vi "Error Handling SubVI Example.vi"(8 "error in (no error)":errorcluster, 10 "Frequency":dbl=10.1, 11 "Amplitude":dbl=1.0) -> (0 "error out":errorcluster, 3 "Waveform":waveform(dbl))   [LabVIEW 2015]
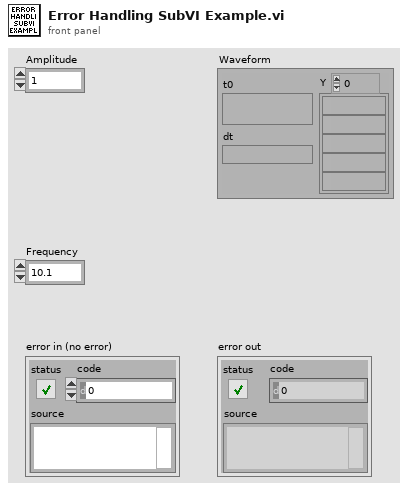
[diagram p1: front panel]
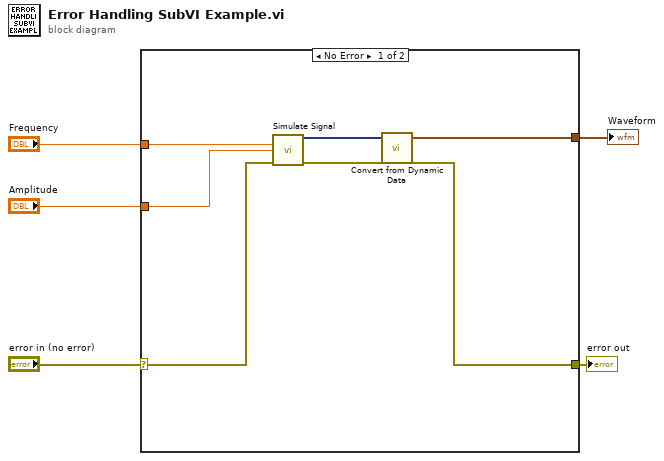
[diagram p0: block diagram]
diagram:
  n1 = case shown="No Error" "error in (no error)" {
    selector: "error in (no error)" -> [w10 w12]
    tunnel: [w9 w12] -> w4
    tunnel: "Frequency" -> [w8 _]
    tunnel: "Amplitude" -> [w7 _]
    tunnel: [w6 _] -> w1
    frame No Error {
      n2 = call "Simulate Signal"("Frequency"=w8, "Amplitude"=w7, "error in (no error)"=w10) -> ("Sine with Uniform Noise"=w11:dynamicdata, "error out"=w9:errorcluster)  [unwired: 11 in]
      n3 = call "Convert from Dynamic Data"("Dynamic Data Type"=w11) -> ("Waveform"=w6:waveform(dbl))  [unwired: 3 in]
    }
    frame Error {
    }
  }
  "error out" <- w4
  "Waveform" <- w1
